vi "simulation.vi"() -> ()   [LabVIEW 2024]
uses:
  <vilib>/Analysis/baseanly.llb/Mean (DBL).vi
  <vilib>/Utility/file.llb/Read Delimited Spreadsheet (DBL).vi
  <vilib>/Analysis/NI_AALBase.lvlib
panel:
  out "x .or. y?":bool
  out "weight_load(ton)":dbl
  out "mean":dbl format="%0.2f"
  out "XY Graph 7":cluster{dbl[], dbl[]}(graph)
  out "XY Graph 6":cluster{dbl[], dbl[]}[](graph)
  out "XY Graph 5":cluster{dbl[], dbl[]}[](graph)
  out "XY Graph 4":cluster{dbl[], dbl[]}[](graph)
  out "XY Graph 3":cluster{dbl[], sgl[]}[](graph)
  out "XY Graph 2":cluster{dbl[], dbl[]}[](graph)
  out "period(Hz)":dbl(knob) scale=0.0..60.0
  out "Histogram Graph":cluster{i32[], u32[]}(graph)
  out "time":dbl format="%.2g"
  out "Slide":dbl(slide) scale=0.0..100.0
  out "error out":errorcluster
  in  "stop":bool
  in  "file path (dialog if empty)":path
  out "XY Graph":cluster{dbl[], dbl[]}(graph)
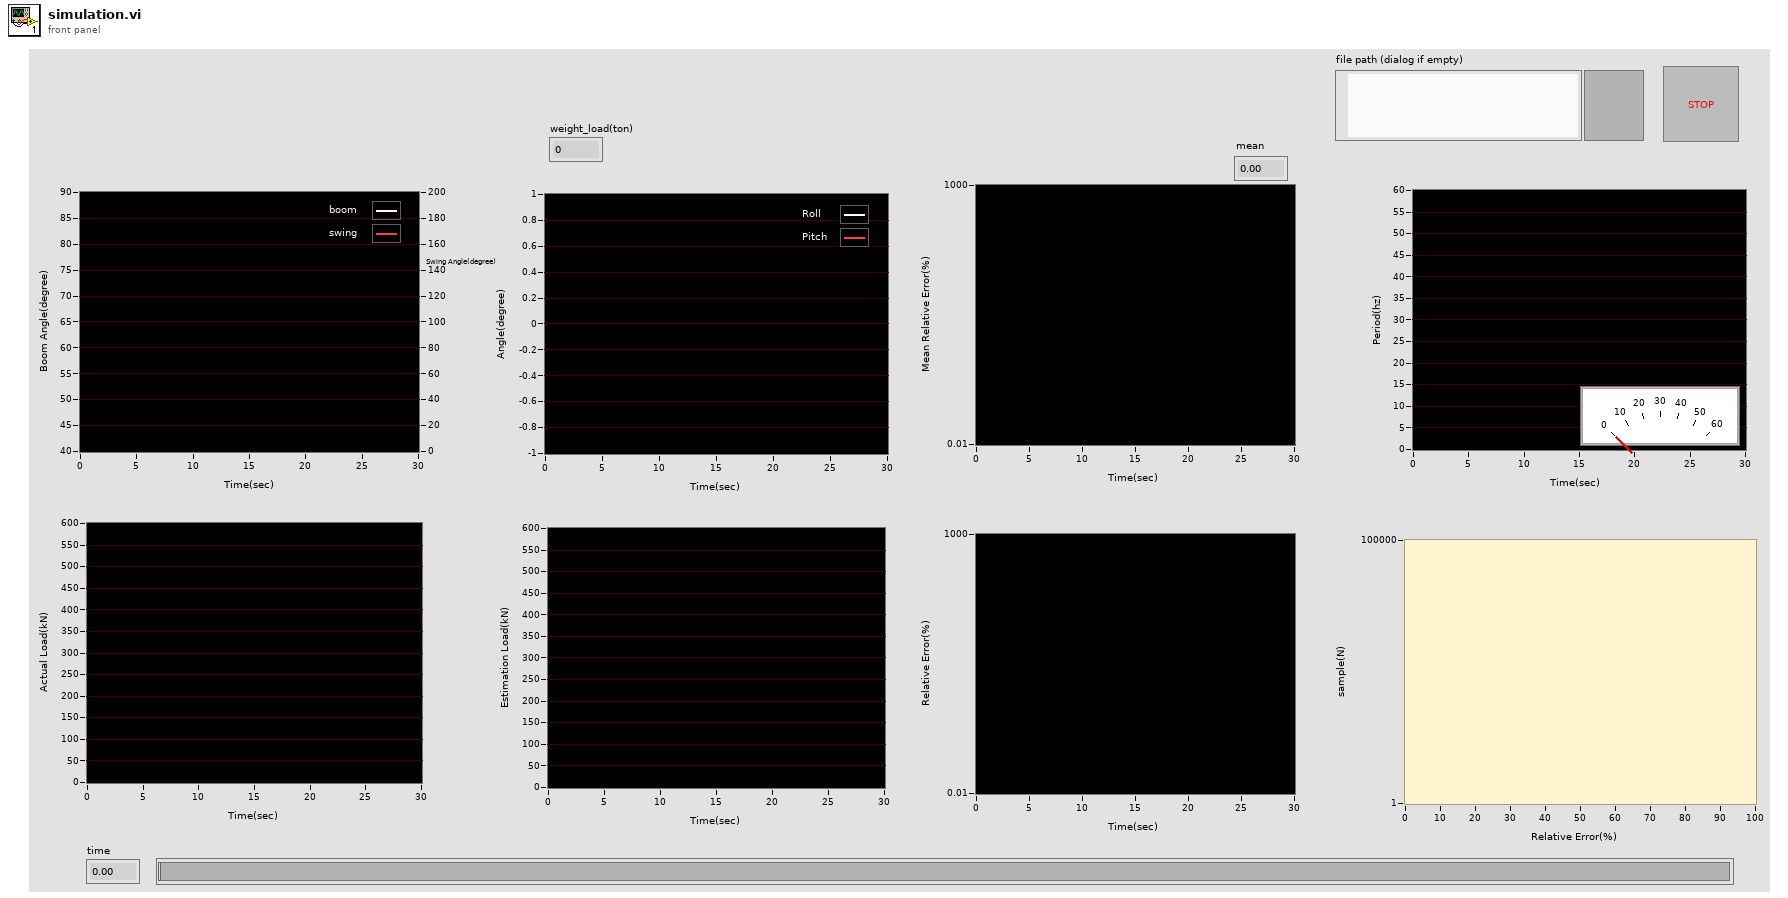
[diagram p1: front panel]
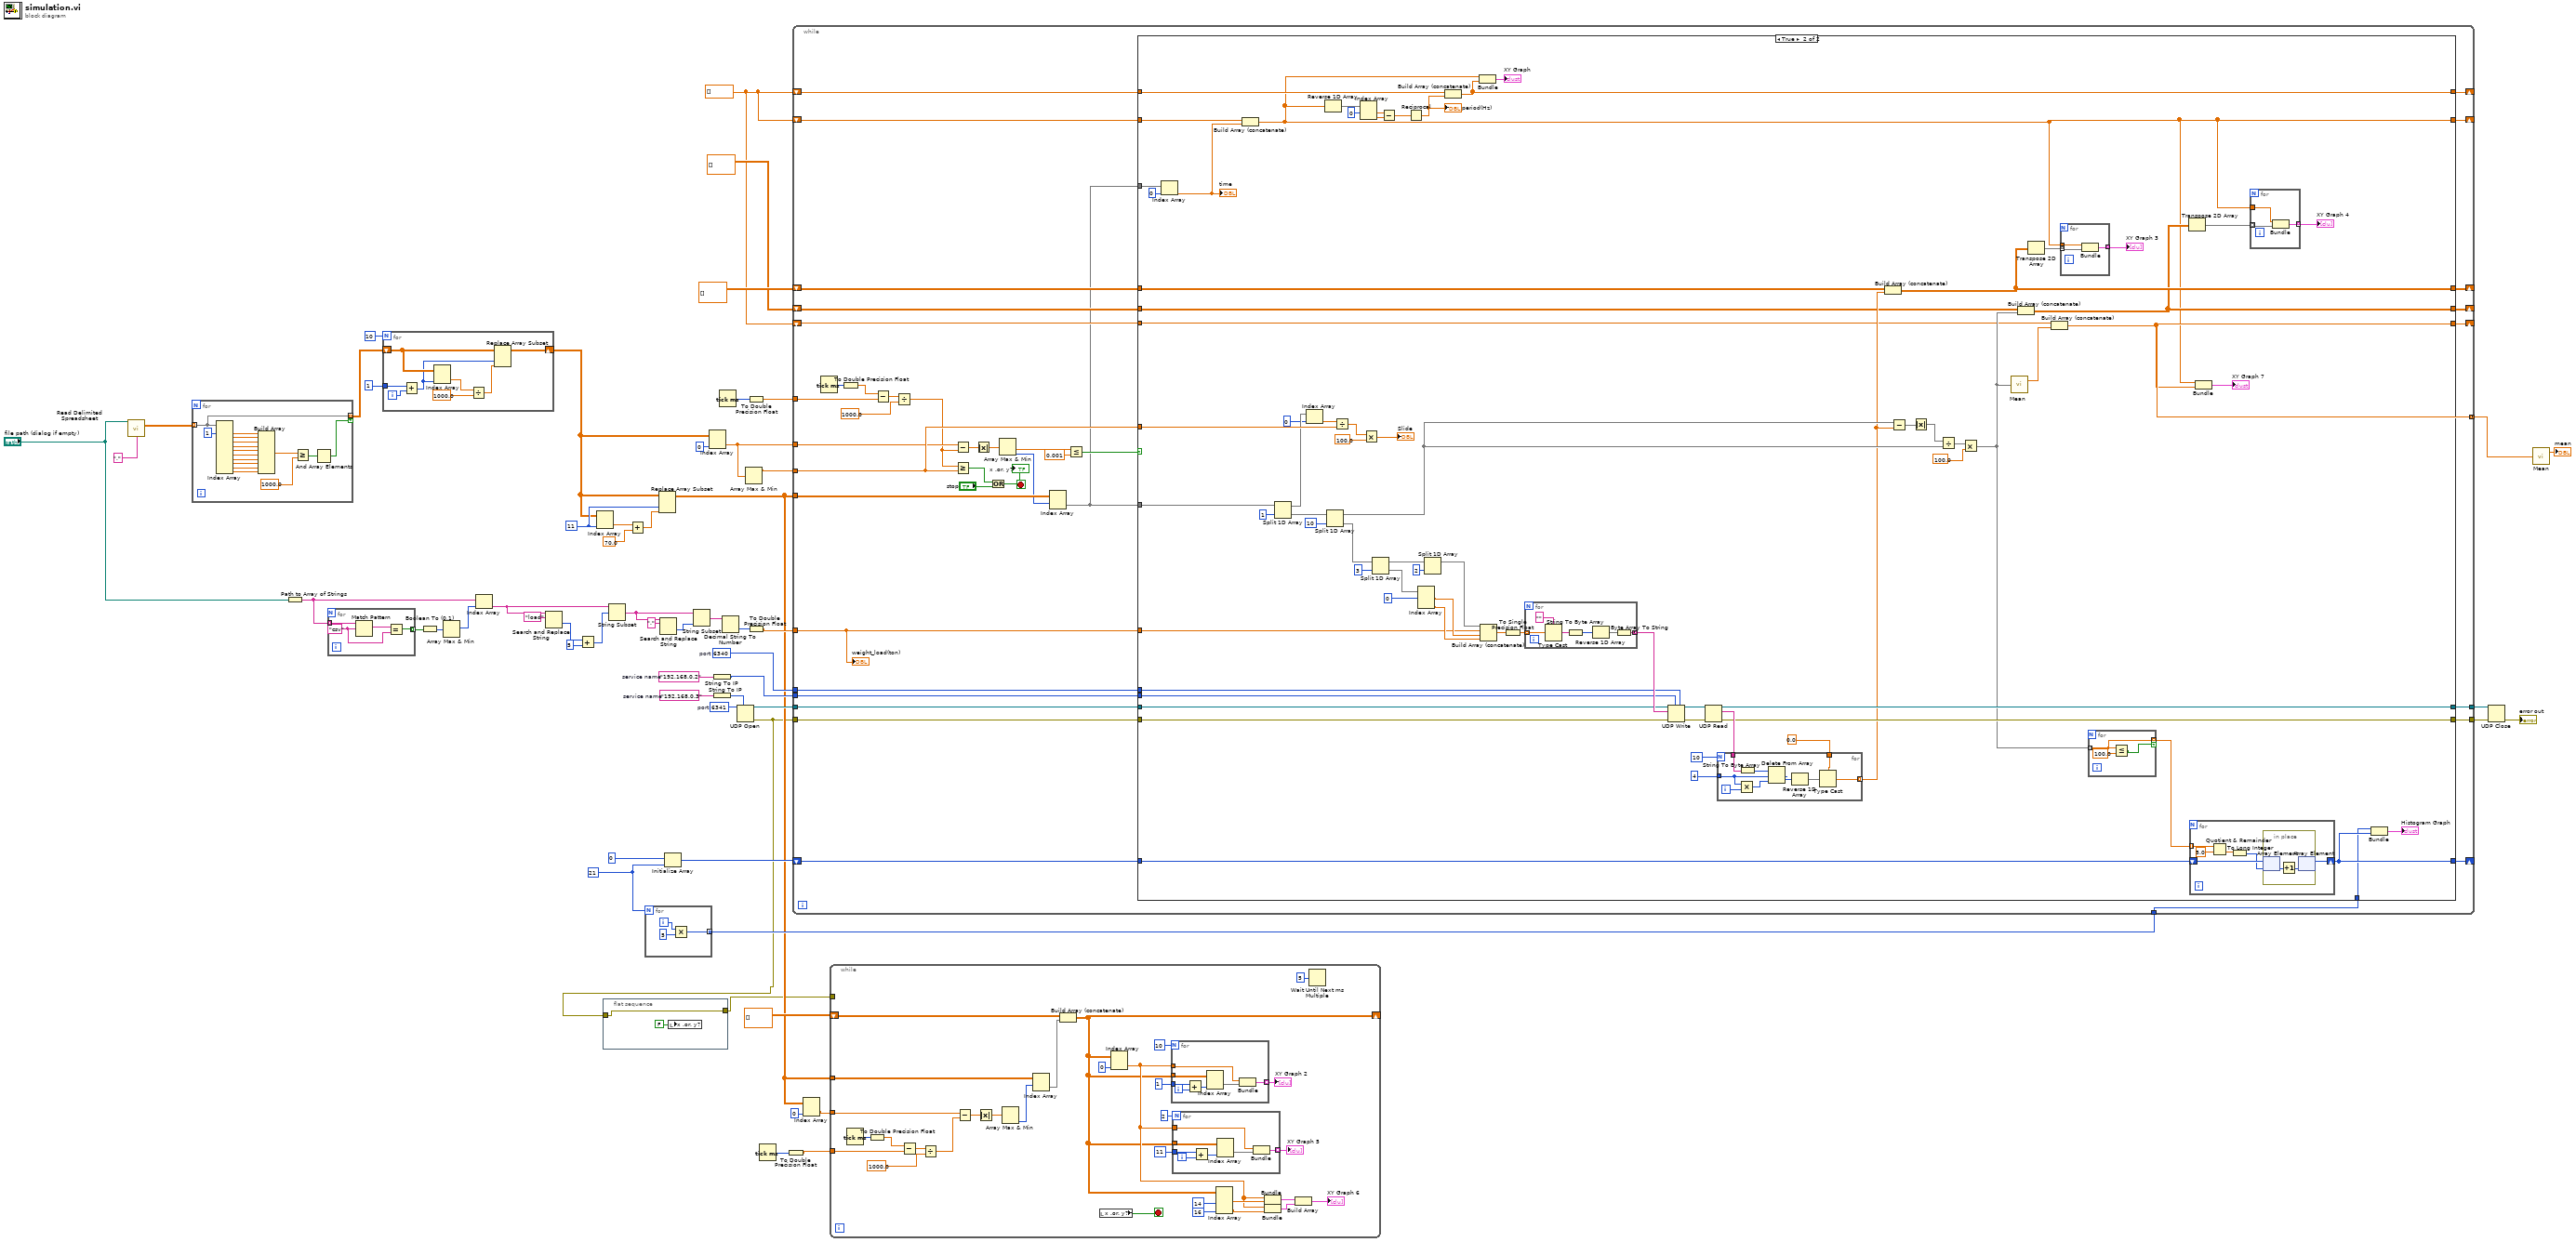
[diagram p0: block diagram]
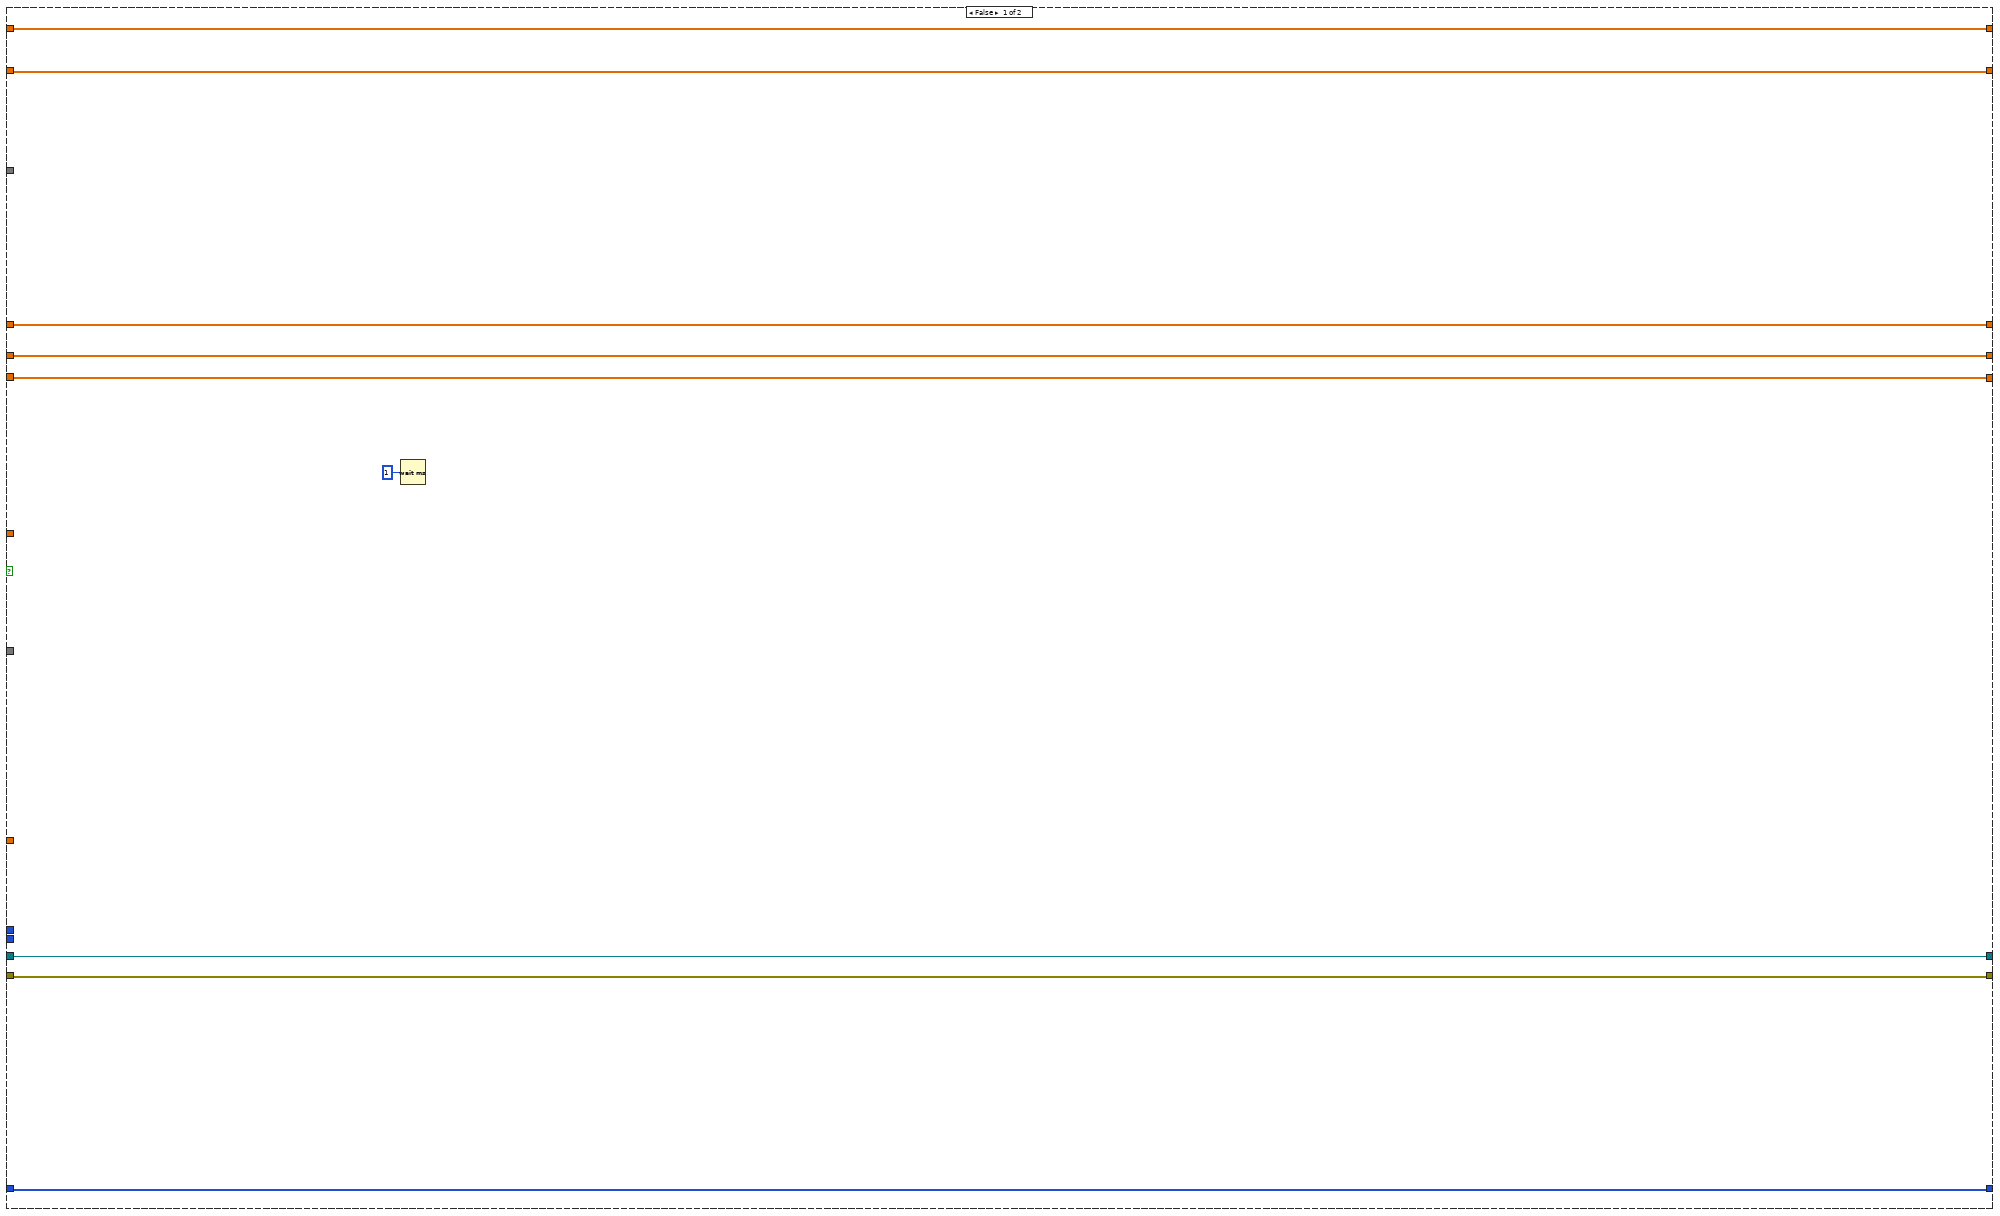
[diagram p2: hidden frame]
diagram:
  w18 = "192.168.0.2"  # service name
  w23 = 11 ("disabled index (col)")
  w10 = dbl[] []
  w43 = 21
  w51 = u16 6340  # port
  w53 = "192.168.0.3"  # service name
  w52 = u16 6341  # port
  n1 = call-poly <vilib>:"Read Delimited Spreadsheet.vi"("file path (dialog if empty)"="file path (dialog if empty)", "delimiter (\\t)"="," ("delimiter (\\t)")) -> ("all rows"=w44:dbl[][])  [unwired: 8 in, 5 out]
  n2 = for {
    tunnel: w44 -> [w60] mode=indexing
    tunnel: [w60] -> w20 mode=indexing if=w59
    n3 = Index Array(array=w60, index #1=1 ("index")) -> (element #1=w73:dbl, element #2=w72:dbl, element #3=w71:dbl, element #4=w70:dbl, element #5=w69:dbl, element #6=w68:dbl, element #7=w67:dbl, element #8=w66:dbl, element #9=w65:dbl, element #10=w64:dbl)  [unwired: 9 in]
    n4 = Build Array(w73, w72, w71, w70, w69, w68, w67, w66, w65, w64) -> (w62:dbl[])
    n5 = Greater Or Equal?(x=w62, y=1000.0) -> (x >= y?=w61:bool[])
    n6 = And Array Elements(Boolean array=w61) -> (logical AND=w59:bool)
  }
  n7 = Path to Array of Strings(0:"file path (dialog if empty)") -> (2:w14:string[])  [unwired: 1 out]
  n8 = for {
    tunnel: w14 -> [w78] mode=indexing
    tunnel: [w75] -> w13 mode=indexing
    w76 = "csv" ("regular expression")
    n9 = Match Pattern(string=w78, regular expression=w76) -> (match substring=w77:string)  [unwired: 1 in, 3 out]
    n10 = Equal?(x=w77, y=w76) -> (x = y?=w75:bool)
  }
  n11 = for {
    N: 10 -> [_]
    tunnel: 1 -> [w86]
    shift-right: [w83] -> w19
    shift-left: w20 -> [w82]
    i -> [w85]
    n12 = Add(x=w86, y=w85) -> (x+y=w79:i32)
    n13 = Index Array(array=w82, index (col)=w79) -> (element=w81:dbl[])  [unwired: 1 in]
    n14 = Divide(x=w81, y=1000.0) -> (x/y=w80:dbl[])
    n15 = Replace Array Subset "Replace Array Subset"(array=w82, new element=w80, index (col)=w79) -> (w83:dbl[][])  [unwired: 1 in]
  }
  n16 = Boolean To (0,1)(Boolean=w13) -> (0, 1=w12:i16[])
  n17 = Array Max & Min(array=w12) -> (max index (indices)=w11:i32)  [unwired: 3 out]
  n18 = Index Array(array=w14, index=w11) -> (element=w30:string)
  n19 = Search and Replace String(input string=w30, search string="load") -> (offset past replacement=w34:i32)  [unwired: 6 in, 3 out]
  n20 = Add(x=w34, y=5) -> (x+y=w35:i32)
  n21 = Index Array(array=w19, index (col)=w23) -> (element=w26:dbl[])  [unwired: 1 in]
  n22 = flat-sequence {
    tunnel: w2 -> [w87]
    tunnel: [w87] -> w1
    frame #0 {
      n23 = local write "x .or. y?"(FALSE ("x .or. y?")) -> ()
    }
  }
  n24 = String Subset(string=w30, offset (0)=w35) -> (substring=w37:string)  [unwired: 1 in]
  n25 = Add(x=w26, y=70.0) -> (x+y=w24:dbl[])
  n26 = for {
    N: w43 -> [_]
    tunnel: [w89] -> w40 mode=indexing
    i -> [w91]
    n27 = Multiply(x=w91, y=5) -> (x*y=w89:i32)
  }
  n28 = Replace Array Subset "Replace Array Subset"(array=w19, new element=w24, index (col)=w23) -> (w5:dbl[][])  [unwired: 1 in]
  n29 = Search and Replace String(input string=w37, search string=".") -> (offset past replacement=w36:i32)  [unwired: 6 in, 3 out]
  n30 = Initialize Array(u32 0 ("y"), w43) -> (w41:u32[])
  n31 = String Subset(string=w37, length (rest)=w36) -> (substring=w38:string)  [unwired: 1 in]
  n32 = Index Array "Index Array"(array=w19, index (col)=0 ("disabled index (col)")) -> (element=w55:dbl[])  [unwired: 1 in]
  n33 = String To IP(1:w18) -> (0:w17:u32)
  n34 = String To IP(1:w53) -> (0:w49:u32)
  n35 = Tick Count (ms)() -> (millisecond timer value=w57:u32)
  n36 = Decimal String To Number(string=w38) -> (number=w39:i32)  [unwired: 2 in, 1 out]
  n37 = UDP Open(7:w49, 11:w52) -> (port=w50:refnum<k16>, 0:w2:errorcluster)  [unwired: 3 in, 1 out]
  n38 = Array Max & Min(array=w55) -> (max value=w54:dbl)  [unwired: 3 out]
  n39 = To Double Precision Float(number=w57) -> (double precision float=w9:dbl)
  n40 = To Double Precision Float(number=w39) -> (double precision float=w29:dbl)
  n41 = Tick Count (ms)() -> (millisecond timer value=w7:u32)
  n42 = To Double Precision Float(number=w7) -> (double precision float=w6:dbl)
  n43 = while {
    tunnel: w9 -> [w129]
    tunnel: w5 -> [w94]
    tunnel: w55 -> [w96]
    tunnel: w54 -> [w116]
    tunnel: w51 -> [w122]
    tunnel: w50 -> [w121]
    tunnel: w2 -> [w120]
    tunnel: w17 -> [w119]
    tunnel: [w118] -> w47
    tunnel: [w117] -> w46
    shift-right: [w114] -> _
    shift-left: w41 -> [w115]
    tunnel: w40 -> [w113]
    shift-right: [w111] -> _
    shift-left: w10 -> [w98]
    tunnel: w29 -> [w112]
    shift-right: [w109] -> _
    shift-left: sgl[][] [] -> [w110]
    shift-right: [w106] -> _
    shift-left: dbl[][] [] -> [w108]
    shift-right: [w105] -> _
    shift-left: w10 -> [w107]
    tunnel: [w105] -> w16 mode=concatenating
    shift-right: [w100] -> _
    shift-left: w10 -> [w101]
    stop <- w97 stop-if-true
    n44 = Tick Count (ms)() -> (millisecond timer value=w130:u32)
    n45 = To Double Precision Float(number=w130) -> (double precision float=w99:dbl)
    n46 = Subtract(x=w99, y=w129) -> (x-y=w128:dbl)
    n47 = Divide(x=w128, y=1000.0) -> (x/y=w95:dbl)
    n48 = Subtract(x=w96, y=w95) -> (x-y=w126:dbl[])
    n49 = Greater Or Equal?(x=w95, y=w116) -> (x >= y?=w123:bool)
    n50 = Absolute Value(x=w126) -> (abs(x)=w125:dbl[])
    n51 = Or(x=w123, y="stop") -> (x .or. y?=w97:bool)
    "x .or. y?" <- w97
    n52 = Array Max & Min(array=w125) -> (min value=w104:dbl, min index (indices)=w93:i32)  [unwired: 2 out]
    n53 = Index Array(array=w94, index (row)=w93) -> (element=w92:dbl[])  [unwired: 1 in]
    n54 = Less Or Equal?(x=w104, y=0.001) -> (x <= y?=w102:bool)
    n55 = case shown="True" w102 {
      tunnel: w122 -> [_ w203]
      tunnel: w121 -> [w136 w202]
      tunnel: w120 -> [w135 w201]
      tunnel: w119 -> [_ w200]
      tunnel: [w136 w193] -> w118
      tunnel: [w135 w192] -> w117
      tunnel: w116 -> [_ w184]
      tunnel: w115 -> [w134 w176]
      tunnel: [w134 w175] -> w114
      tunnel: w113 -> [_ w174]
      tunnel: w112 -> [_ w172]
      tunnel: [w132 w150] -> w111
      tunnel: w110 -> [w139 w170]
      tunnel: [w139 w168] -> w109
      tunnel: w108 -> [w138 w165]
      tunnel: w107 -> [w137 w158]
      tunnel: [w138 w156] -> w106
      tunnel: [w137 w154] -> w105
      tunnel: w92 -> [_ w153]
      tunnel: w101 -> [w133 w152]
      tunnel: [w133 w149] -> w100
      tunnel: w98 -> [w132 w151]
      tunnel: w92 -> [_ w141]
      frame False {
        n56 = Wait (ms)(milliseconds to wait=u32 1) -> ()  [unwired: 1 out]
      }
      frame True {
        n57 = Index Array(array=w141, index=0) -> (element=w142:dbl)
        "time" <- w142
        n58 = Build Array (concatenate)(w152, w142) -> (w149:dbl[])
        n59 = Split 1D Array(array=w153, index=1) -> (first subarray=w183:dbl[], second subarray=w211:dbl[])
        n60 = Index Array(array=w183, index=0) -> (element=w181:dbl)
        n61 = Reverse 1D Array(array=w149) -> (reversed array=w148:dbl[])
        n62 = Split 1D Array(array=w211, index=10) -> (first subarray=w208:dbl[], second subarray=w209:dbl[])
        n63 = Divide(x=w181, y=w184) -> (x/y=w180:dbl)
        n64 = Index Array(array=w148, index #1=0 ("index")) -> (element #1=w145:dbl, element #2=w146:dbl)  [unwired: 1 in]
        n65 = Multiply(x=w180, y=100.0) -> (x*y=→"Slide":dbl)
        n66 = Split 1D Array(array=w209, index=3) -> (first subarray=w161:dbl[], second subarray=w207:dbl[])
        n67 = Subtract(x=w145, y=w146) -> (x-y=w144:dbl)
        n68 = Reciprocal(x=w144) -> (1/x=w143:dbl)
        "period(Hz)" <- w143
        n69 = Index Array(array=w207, index #1=0 ("index")) -> (element #1=w191:dbl, element #3=w190:dbl)  [unwired: 2 in, 1 out]
        n70 = Split 1D Array(array=w161, index=2) -> (first subarray=w159:dbl[])  [unwired: 1 out]
        n71 = Build Array (concatenate)(w151, w143) -> (w150:dbl[])
        n72 = Bundle(w149, w150) -> (→"XY Graph":cluster{dbl[], dbl[]})  [unwired: 1 in]
        n73 = Build Array (concatenate)(w159, w172, w191, w190) -> (w205:dbl[])
        n74 = To Single Precision Float(number=w205) -> (single precision float=w189:sgl[])
        n75 = for {
          tunnel: w189 -> [w237] mode=indexing
          tunnel: [w232] -> w204 mode=concatenating
          n76 = Type Cast(type="" ("data out"), x=w237) -> (*(type *) &x=w235:string)
          n77 = String To Byte Array(string=w235) -> (unsigned byte array=w234:u8[])
          n78 = Reverse 1D Array(array=w234) -> (reversed array=w233:u8[])
          n79 = Byte Array To String(unsigned byte array=w233) -> (string=w232:string)
        }
        n80 = UDP Write(address=w200, port or service name=w203, connection ID=w202, data in=w204, 8:w201) -> (error out=w195:errorcluster, 3:w196:refnum<k16>)  [unwired: 1 in]
        n81 = UDP Read(connection ID=w196, 8:w195) -> (data out=w194:string, error out=w192:errorcluster, 3:w193:refnum<k16>)  [unwired: 2 in, 2 out]
        n82 = for {
          N: 10 -> [_]
          tunnel: w194 -> [w231]
          tunnel: 4 ("length") -> [w228]
          tunnel: sgl 0.0 -> [w224]
          tunnel: [w223] -> w169 mode=indexing
          i -> [w229]
          n83 = Multiply(x=w228, y=w229) -> (x*y=w227:i32)
          n84 = String To Byte Array(string=w231) -> (unsigned byte array=w230:u8[])
          n85 = Delete From Array(array=w230, length=w228, index=w227) -> (deleted portion=w226:u8[])  [unwired: 1 out]
          n86 = Reverse 1D Array(array=w226) -> (reversed array=w225:u8[])
          n87 = Type Cast(type=w224, x=w225) -> (*(type *) &x=w223:sgl)
        }
        n88 = Build Array (concatenate)(w170, w169) -> (w168:sgl[][])
        n89 = Subtract(x=w208, y=w169) -> (x-y=w188:dbl[])
        n90 = Absolute Value(x=w188) -> (abs(x)=w187:dbl[])
        n91 = Divide(x=w187, y=w208) -> (x/y=w186:dbl[])
        n92 = Multiply(x=w186, y=100.0) -> (x*y=w164:dbl[])
        n93 = call-poly <vilib>:"Mean.vi"("X"=w164) -> ("mean"=w157:dbl)  [unwired: 1 out]
        n94 = Build Array (concatenate)(w165, w164) -> (w156:dbl[][])
        n95 = Transpose 2D Array(2D array=w168) -> (transposed array=w167:sgl[][])
        n96 = Build Array (concatenate)(w158, w157) -> (w154:dbl[])
        n97 = for {
          tunnel: w149 -> [w219]
          tunnel: [w218] -> w166 mode=indexing
          tunnel: w167 -> [w217] mode=indexing
          n98 = Bundle(w219, w217) -> (w218:cluster{dbl[], sgl[]})  [unwired: 1 in]
        }
        "XY Graph 3" <- w166
        n99 = for {
          tunnel: w164 -> [w221] mode=indexing
          tunnel: [w221] -> w173 mode=indexing if=w220
          n100 = Less Or Equal?(x=w221, y=100.0) -> (x <= y?=w220:bool)
        }
        n101 = Transpose 2D Array(2D array=w156) -> (transposed array=w162:dbl[][])
        n102 = for {
          tunnel: w173 -> [w240] mode=indexing
          shift-right: [w242] -> w175
          shift-left: w176 -> [w243]
          n103 = Quotient & Remainder(x=w240, y=5.0) -> (floor(x/y)=w239:dbl)  [unwired: 1 out]
          n104 = To Long Integer(number=w239) -> (32bit integer=w238:i32)
          n105 = in-place {
            n106 = in-place-array #1(w243, w238) -> (w245:u32)
            n107 = Increment(x=w245) -> (x+1=w244:u32)
            n108 = in-place-array #1(w244) -> (w242:u32[])  [unwired: 1 out]
          }
        }
        n109 = Bundle(w149, w154) -> (→"XY Graph 7":cluster{dbl[], dbl[]})  [unwired: 1 in]
        n110 = for {
          tunnel: w149 -> [w216]
          tunnel: [w215] -> w163 mode=indexing
          tunnel: w162 -> [w214] mode=indexing
          n111 = Bundle(w216, w214) -> (w215:cluster{dbl[], dbl[]})  [unwired: 1 in]
        }
        "XY Graph 4" <- w163
        n112 = Bundle(w174, w175) -> (→"Histogram Graph":cluster{i32[], u32[]})  [unwired: 1 in]
      }
    }
    "weight_load(ton)" <- w112
  }
  n113 = Index Array(array=w5, index (col)=0 ("disabled index (col)")) -> (element=w3:dbl[])  [unwired: 1 in]
  n114 = while {
    tunnel: w1 -> [_]
    tunnel: w5 -> [w264]
    shift-right: [w246] -> _
    shift-left: dbl[][] [] -> [w268]
    tunnel: w6 -> [w269]
    tunnel: w3 -> [w260]
    stop <- w276 stop-if-true
    n115 = Tick Count (ms)() -> (millisecond timer value=w273:u32)
    n116 = To Double Precision Float(number=w273) -> (double precision float=w270:dbl)
    n117 = Subtract(x=w270, y=w269) -> (x-y=w272:dbl)
    n118 = Divide(x=w272, y=1000.0) -> (x/y=w259:dbl)
    n119 = Subtract(x=w260, y=w259) -> (x-y=w262:dbl[])
    n120 = Absolute Value(x=w262) -> (abs(x)=w261:dbl[])
    n121 = Array Max & Min(array=w261) -> (min index (indices)=w258:i32)  [unwired: 3 out]
    n122 = Index Array(array=w264, index (row)=w258) -> (element=w263:dbl[])  [unwired: 1 in]
    n123 = Build Array (concatenate)(w268, w263) -> (w246:dbl[][])
    n124 = local read "x .or. y?"() -> (w276:bool)
    n125 = Index Array(array=w246, index (col)=0 ("disabled index (col)")) -> (element=w247:dbl[])  [unwired: 1 in]
    n126 = for {
      N: 10 -> [_]
      tunnel: w246 -> [w290]
      tunnel: w247 -> [w289]
      tunnel: 1 -> [w288]
      tunnel: [w285] -> w275 mode=indexing
      i -> [w287]
      n127 = Add(x=w288, y=w287) -> (x+y=w286:i32)
      n128 = Index Array(array=w290, index (col)=w286) -> (element=w284:dbl[])  [unwired: 1 in]
      n129 = Bundle(w289, w284) -> (w285:cluster{dbl[], dbl[]})  [unwired: 1 in]
    }
    "XY Graph 2" <- w275
    n130 = for {
      N: 2 -> [_]
      tunnel: w246 -> [w283]
      tunnel: w247 -> [w282]
      tunnel: 11 -> [w281]
      tunnel: [w278] -> w257 mode=indexing
      i -> [w280]
      n131 = Add(x=w281, y=w280) -> (x+y=w279:i32)
      n132 = Index Array(array=w283, index (col)=w279) -> (element=w277:dbl[])  [unwired: 1 in]
      n133 = Bundle(w282, w277) -> (w278:cluster{dbl[], dbl[]})  [unwired: 1 in]
    }
    "XY Graph 5" <- w257
    n134 = Index Array(array=w246, index (col) #1=14 ("disabled index (col)"), index (col) #2=16 ("disabled index (col)")) -> (element #1=w253:dbl[], element #2=w254:dbl[])  [unwired: 2 in]
    n135 = Bundle(w247, w253) -> (w250:cluster{dbl[], dbl[]})  [unwired: 1 in]
    n136 = Bundle(w247, w254) -> (w251:cluster{dbl[], dbl[]})  [unwired: 1 in]
    n137 = Build Array(w250, w251) -> (→"XY Graph 6":cluster{dbl[], dbl[]}[])
    n138 = Wait Until Next ms Multiple(millisecond multiple=u32 5) -> ()  [unwired: 1 out]
  }
  n139 = UDP Close(connection ID=w47, 8:w46) -> (error out=→"error out":errorcluster)  [unwired: 1 out]
  n140 = call-poly <vilib>:"Mean.vi"("X"=w16) -> ("mean"=→"mean":dbl)  [unwired: 1 out]
